vi "二型板自动测试合格率统计.vi"() -> ()   [LabVIEW 2010]
uses:
  全局量/试验配置信息.vi
  全局量/自动测试结果.vi
panel:
  in  "自测序号":i32
  in  "自测类型4合格路数":i32
  in  "自测类型3合格路数":i32
  in  "自测类型2合格路数":i32
  in  "自测类型1合格路数":i32
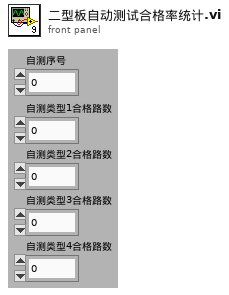
[diagram p1: front panel]
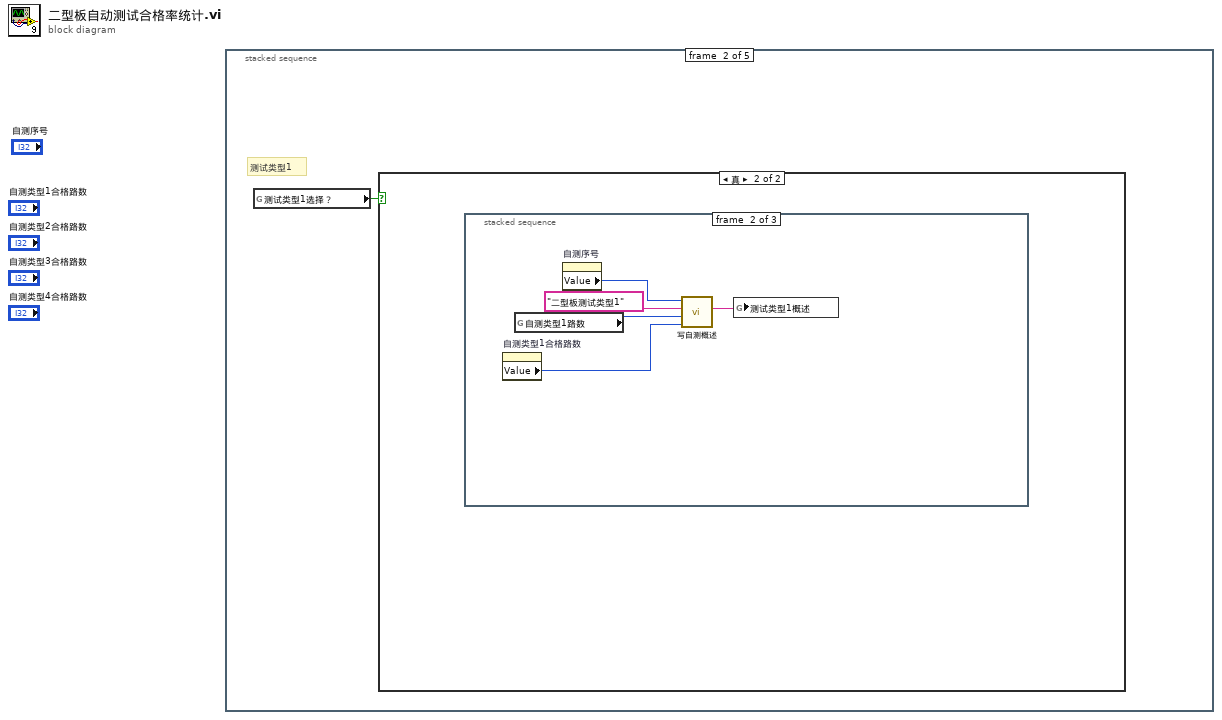
[diagram p0: block diagram]
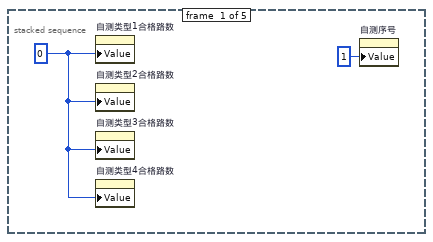
[diagram p2: hidden frame]
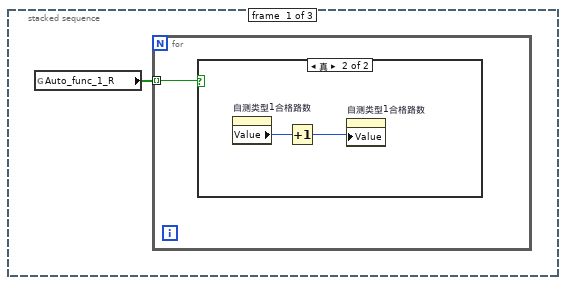
[diagram p4: hidden frame]
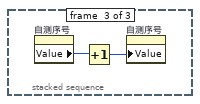
[diagram p6: hidden frame]
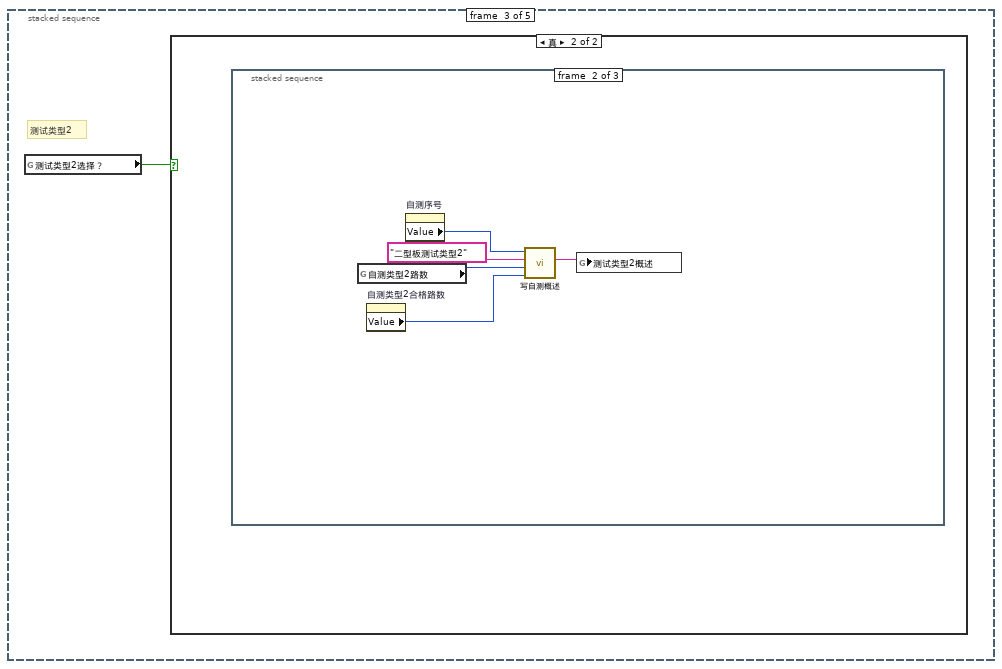
[diagram p7: hidden frame]
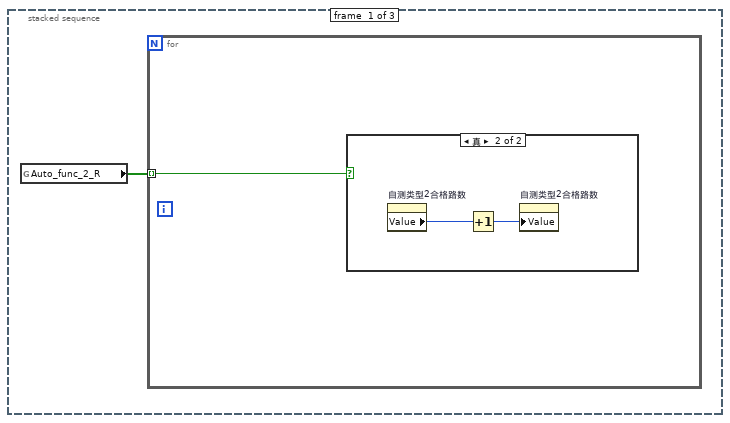
[diagram p9: hidden frame]
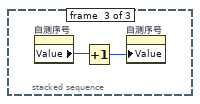
[diagram p11: hidden frame]
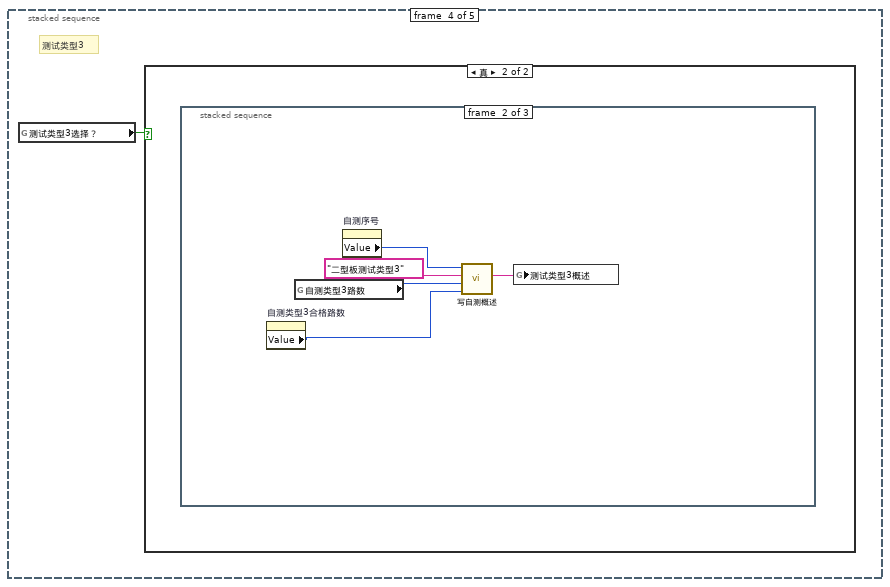
[diagram p12: hidden frame]
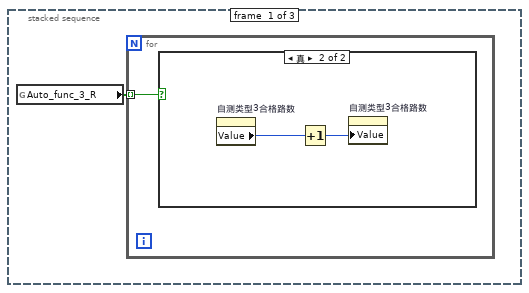
[diagram p14: hidden frame]
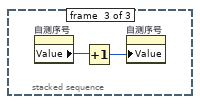
[diagram p16: hidden frame]
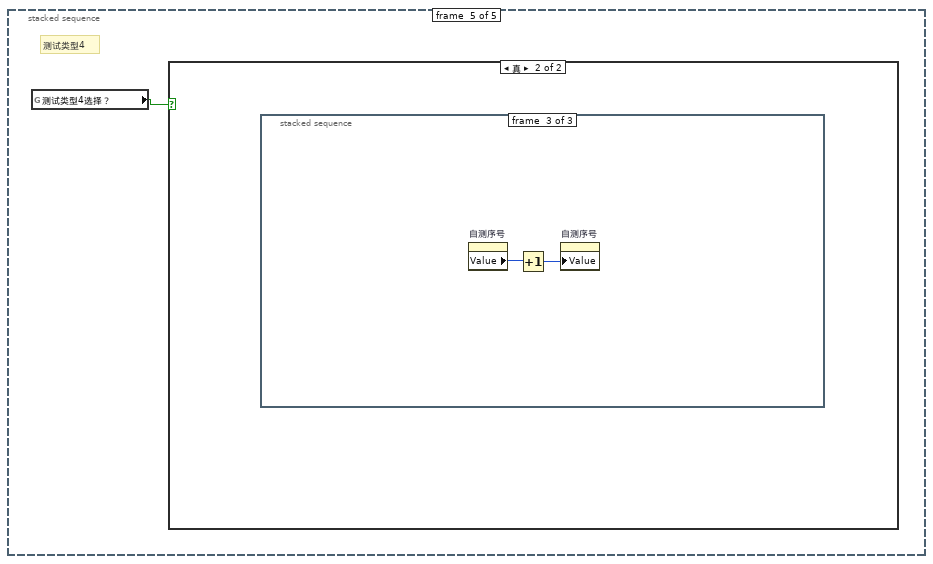
[diagram p17: hidden frame]
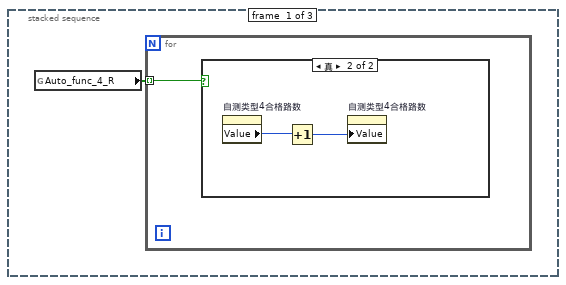
[diagram p19: hidden frame]
diagram:
  n1 = stacked-sequence {
    frame #0 {
      w2 = 0 ("数字量输入合格路数")
      n2 = property on="自测类型1合格路数" class="DigNum (严格)"("Value"=w2) -> ()  [unwired: 2 in, 2 out]
      n3 = property on="自测类型2合格路数" class="DigNum (严格)"("Value"=w2) -> ()  [unwired: 2 in, 2 out]
      n4 = property on="自测类型3合格路数" class="DigNum (严格)"("Value"=w2) -> ()  [unwired: 2 in, 2 out]
      n5 = property on="自测类型4合格路数" class="DigNum (严格)"("Value"=w2) -> ()  [unwired: 2 in, 2 out]
      n6 = property on="自测序号" class="DigNum (严格)"("Value"=1 ("自测序号")) -> ()  [unwired: 2 in, 2 out]
    }
    frame #1 {
      # "测试类型1"
      n7 = global read "试验配置信息.vi" "测试类型1选择？"() -> (w3:bool)
      n8 = case shown="真" w3 {
        frame False {
        }
        frame True {
          n9 = stacked-sequence {
            frame #0 {
              n10 = global read "自动测试结果.vi" "Auto_func_1_R"() -> (w4:bool[])
              n11 = for {
                tunnel: w4 -> [w5] mode=indexing
                n12 = case shown="真" w5 {
                  frame False {
                  }
                  frame True {
                    n13 = property on="自测类型1合格路数" class="DigNum (严格)"() -> ("Value"=w6:i32)  [unwired: 2 in, 2 out]
                    n14 = Increment(x=w6) -> (x+1=w7:i32)
                    n15 = property on="自测类型1合格路数" class="DigNum (严格)"("Value"=w7) -> ()  [unwired: 2 in, 2 out]
                  }
                }
              }
            }
            frame #1 {
              n16 = property on="自测类型1合格路数" class="DigNum (严格)"() -> ("Value"=w9:i32)  [unwired: 2 in, 2 out]
              n17 = global read "试验配置信息.vi" "自测类型1路数"() -> (w10:i32)
              n18 = property on="自测序号" class="DigNum (严格)"() -> ("Value"=w12:i32)  [unwired: 2 in, 2 out]
              n19 = call "写自测概述.vi"("合格路数"=w9, "共路数"=w10, "测试事项"="二型板测试类型1", "自测序号"=w12) -> ("概述字符串"=w8:string)  [unwired: 7 in]
              n20 = global write "自动测试结果.vi" "测试类型1概述"(w8) -> ()
            }
            frame #2 {
              n21 = property on="自测序号" class="DigNum (严格)"() -> ("Value"=w13:i32)  [unwired: 2 in, 2 out]
              n22 = Increment(x=w13) -> (x+1=w14:i32)
              n23 = property on="自测序号" class="DigNum (严格)"("Value"=w14) -> ()  [unwired: 2 in, 2 out]
            }
          }
        }
      }
    }
    frame #2 {
      # "测试类型2"
      n24 = global read "试验配置信息.vi" "测试类型2选择？"() -> (w15:bool)
      n25 = case shown="真" w15 {
        frame False {
        }
        frame True {
          n26 = stacked-sequence {
            frame #0 {
              n27 = global read "自动测试结果.vi" "Auto_func_2_R"() -> (w16:bool[])
              n28 = for {
                tunnel: w16 -> [w17] mode=indexing
                n29 = case shown="真" w17 {
                  frame False {
                  }
                  frame True {
                    n30 = property on="自测类型2合格路数" class="DigNum (严格)"() -> ("Value"=w18:i32)  [unwired: 2 in, 2 out]
                    n31 = Increment(x=w18) -> (x+1=w19:i32)
                    n32 = property on="自测类型2合格路数" class="DigNum (严格)"("Value"=w19) -> ()  [unwired: 2 in, 2 out]
                  }
                }
              }
            }
            frame #1 {
              n33 = global read "试验配置信息.vi" "自测类型2路数"() -> (w24:i32)
              n34 = property on="自测类型2合格路数" class="DigNum (严格)"() -> ("Value"=w21:i32)  [unwired: 2 in, 2 out]
              n35 = property on="自测序号" class="DigNum (严格)"() -> ("Value"=w22:i32)  [unwired: 2 in, 2 out]
              n36 = call "写自测概述.vi"("合格路数"=w21, "共路数"=w24, "测试事项"="二型板测试类型2", "自测序号"=w22) -> ("概述字符串"=w20:string)  [unwired: 7 in]
              n37 = global write "自动测试结果.vi" "测试类型2概述"(w20) -> ()
            }
            frame #2 {
              n38 = property on="自测序号" class="DigNum (严格)"() -> ("Value"=w26:i32)  [unwired: 2 in, 2 out]
              n39 = Increment(x=w26) -> (x+1=w25:i32)
              n40 = property on="自测序号" class="DigNum (严格)"("Value"=w25) -> ()  [unwired: 2 in, 2 out]
            }
          }
        }
      }
    }
    frame #3 {
      # "测试类型3"
      n41 = global read "试验配置信息.vi" "测试类型3选择？"() -> (w27:bool)
      n42 = case shown="真" w27 {
        frame False {
        }
        frame True {
          n43 = stacked-sequence {
            frame #0 {
              n44 = global read "自动测试结果.vi" "Auto_func_3_R"() -> (w28:bool[])
              n45 = for {
                tunnel: w28 -> [w29] mode=indexing
                n46 = case shown="真" w29 {
                  frame False {
                  }
                  frame True {
                    n47 = property on="自测类型3合格路数" class="DigNum (严格)"() -> ("Value"=w30:i32)  [unwired: 2 in, 2 out]
                    n48 = Increment(x=w30) -> (x+1=w31:i32)
                    n49 = property on="自测类型3合格路数" class="DigNum (严格)"("Value"=w31) -> ()  [unwired: 2 in, 2 out]
                  }
                }
              }
            }
            frame #1 {
              n50 = property on="自测类型3合格路数" class="DigNum (严格)"() -> ("Value"=w32:i32)  [unwired: 2 in, 2 out]
              n51 = global read "试验配置信息.vi" "自测类型3路数"() -> (w35:i32)
              n52 = property on="自测序号" class="DigNum (严格)"() -> ("Value"=w33:i32)  [unwired: 2 in, 2 out]
              n53 = call "写自测概述.vi"("合格路数"=w32, "共路数"=w35, "测试事项"="二型板测试类型3", "自测序号"=w33) -> ("概述字符串"=w36:string)  [unwired: 7 in]
              n54 = global write "自动测试结果.vi" "测试类型3概述"(w36) -> ()
            }
            frame #2 {
              n55 = property on="自测序号" class="DigNum (严格)"() -> ("Value"=w37:i32)  [unwired: 2 in, 2 out]
              n56 = Increment(x=w37) -> (x+1=w38:i32)
              n57 = property on="自测序号" class="DigNum (严格)"("Value"=w38) -> ()  [unwired: 2 in, 2 out]
            }
          }
        }
      }
    }
    frame #4 {
      # "测试类型4"
      n58 = global read "试验配置信息.vi" "测试类型4选择？"() -> (w39:bool)
      n59 = case shown="真" w39 {
        frame False {
        }
        frame True {
          n60 = stacked-sequence {
            frame #0 {
              n61 = global read "自动测试结果.vi" "Auto_func_4_R"() -> (w40:bool[])
              n62 = for {
                tunnel: w40 -> [w41] mode=indexing
                n63 = case shown="真" w41 {
                  frame False {
                  }
                  frame True {
                    n64 = property on="自测类型4合格路数" class="DigNum (严格)"() -> ("Value"=w43:i32)  [unwired: 2 in, 2 out]
                    n65 = Increment(x=w43) -> (x+1=w42:i32)
                    n66 = property on="自测类型4合格路数" class="DigNum (严格)"("Value"=w42) -> ()  [unwired: 2 in, 2 out]
                  }
                }
              }
            }
            frame #1 {
              n67 = global read "试验配置信息.vi" "自测类型4路数"() -> (w46:i32)
              n68 = property on="自测类型4合格路数" class="DigNum (严格)"() -> ("Value"=w44:i32)  [unwired: 2 in, 2 out]
              n69 = property on="自测序号" class="DigNum (严格)"() -> ("Value"=w48:i32)  [unwired: 2 in, 2 out]
              n70 = call "写自测概述.vi"("合格路数"=w44, "共路数"=w46, "测试事项"="二型板测试类型4", "自测序号"=w48) -> ("概述字符串"=w45:string)  [unwired: 7 in]
              n71 = global write "自动测试结果.vi" "测试类型4概述"(w45) -> ()
            }
            frame #2 {
              n72 = property on="自测序号" class="DigNum (严格)"() -> ("Value"=w49:i32)  [unwired: 2 in, 2 out]
              n73 = Increment(x=w49) -> (x+1=w50:i32)
              n74 = property on="自测序号" class="DigNum (严格)"("Value"=w50) -> ()  [unwired: 2 in, 2 out]
            }
          }
        }
      }
    }
  }
